vi "Read Values.vi"(8 "error in":errorcluster, 11 "Report Viewer in":refnum<class "Report Viewer.lvclass">) -> (0 "error out":errorcluster, 3 "Report Viewer out":refnum<class "Report Viewer.lvclass">)   [LabVIEW 2019, in "Report Viewer.lvlib" / "Report Viewer.lvclass"]
uses:
  Library/Report Viewer.lvclass
  Library/Report Viewer.lvclass/Report Viewer.ctl
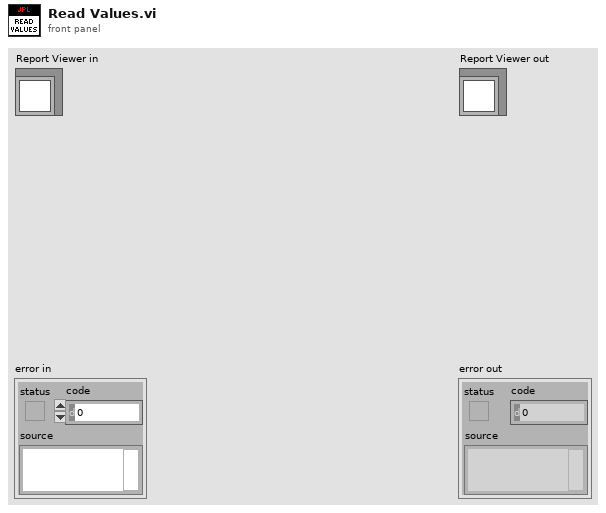
[diagram p1: front panel]
types:
  T1 = typedef "Report Viewer.lvlib/Report Viewer.lvclass/Data to Read.ctl" = cluster{"Group":string, "Channel":string}
  T2 = typedef "Report Viewer.lvlib/Report Viewer.lvclass/Load Method.ctl" = enum16{"Number of Values", "By Time"}
  T3 = typedef "Report Viewer.lvlib/Report Viewer.lvclass/Channel_Timing.ctl" = cluster{"Data Type":u16, "Channel Length":u64, "wf_start_time":timestamp, "wf_increment":dbl}
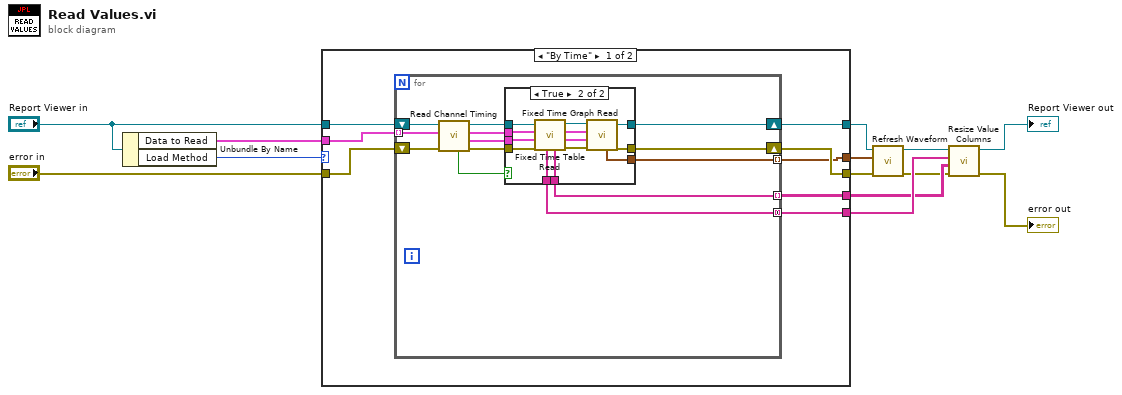
[diagram p0: block diagram]
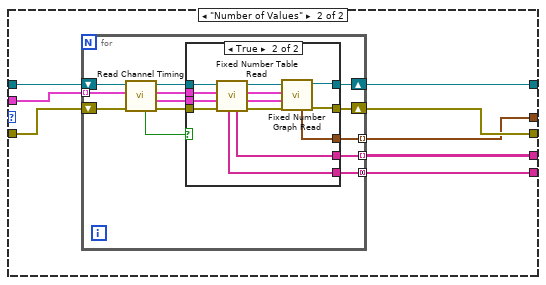
[diagram p3: hidden frame]
diagram:
  n1 = Unbundle By Name("Report Viewer in") -> ("Data to Read"=w9:T1[], "Load Method"=w8:T2)
  n2 = case shown="\"By Time\"" w8 {
    tunnel: [w21 w52] -> w2
    tunnel: [w20 w51] -> w3
    tunnel: "error in" -> [w19 w57]
    tunnel: "Report Viewer in" -> [w18 w56]
    tunnel: w9 -> [w17 w55]
    tunnel: [w15 w54] -> w6
    tunnel: [w16 w53] -> w7
    tunnel: [w14 w50] -> w1
    frame "By Time" {
      n3 = for {
        shift-right: [w34] -> w21
        shift-left: w18 -> [w32]
        shift-right: [w33] -> w20
        shift-left: w19 -> [w28]
        tunnel: w17 -> [w27] mode=indexing
        tunnel: [w24] -> w16 mode=concatenating
        tunnel: [w23] -> w15 mode=indexing
        tunnel: [w22] -> w14 mode=indexing
        n4 = call "Read Channel Timing.vi"("error in"=w28, "Data to read in"=w27, "Report Viewer in"=w32) -> ("error out"=w30:errorcluster, "Data to read out"=w25:T1, "Channel_Timing"=w29:T3, "Report Viewer out"=w31:refnum<class "Report Viewer.lvclass">, "Good_Record"=w26:bool)  [unwired: 4 in]
        n5 = case shown="True" w26 {
          tunnel: [w35 w40] -> w34
          tunnel: [w36 w41] -> w33
          tunnel: w31 -> [w35 w49]
          tunnel: w30 -> [w36 w48]
          tunnel: w29 -> [_ w47]
          tunnel: w25 -> [_ w46]
          tunnel: [_ w45] -> w24
          tunnel: [_ w44] -> w23
          tunnel: [_ w37] -> w22
          frame False {
          }
          frame True {
            n6 = call "Fixed Time Table Read.vi"("error in"=w48, "Data to read in"=w46, "Channel_Timing in"=w47, "Report Viewer in"=w49) -> ("error out"=w42:errorcluster, "Data to read out"=w38:T1, "Channel_Timing out"=w39:T3, "Report Viewer out"=w43:refnum<class "Report Viewer.lvclass">, "Table Data"=w44:string[], "Table_Header"=w45:string[])  [unwired: 2 in]
            n7 = call "Fixed Time Graph Read.vi"("error in"=w42, "Data to read in"=w38, "Channel_Timing in"=w39, "Report Viewer in"=w43) -> ("error out"=w41:errorcluster, "Report Viewer out"=w40:refnum<class "Report Viewer.lvclass">, "Waveform"=w37:waveform(dbl))  [unwired: 3 in, 2 out]
          }
        }
      }
    }
    frame "Number of Values" {
      n8 = for {
        shift-right: [w65] -> w52
        shift-left: w56 -> [w70]
        shift-right: [w64] -> w51
        shift-left: w57 -> [w69]
        tunnel: w55 -> [w68] mode=indexing
        tunnel: [w60] -> w54 mode=indexing
        tunnel: [w59] -> w53 mode=concatenating
        tunnel: [w58] -> w50 mode=indexing
        n9 = call "Read Channel Timing.vi"("error in"=w69, "Data to read in"=w68, "Report Viewer in"=w70) -> ("error out"=w67:errorcluster, "Data to read out"=w61:T1, "Channel_Timing"=w63:T3, "Report Viewer out"=w66:refnum<class "Report Viewer.lvclass">, "Good_Record"=w62:bool)  [unwired: 4 in]
        n10 = case shown="True" w62 {
          tunnel: w67 -> [w71 w81]
          tunnel: w66 -> [w72 w80]
          tunnel: [w72 w84] -> w65
          tunnel: [w71 w85] -> w64
          tunnel: w63 -> [_ w79]
          tunnel: w61 -> [_ w78]
          tunnel: [_ w75] -> w60
          tunnel: [_ w74] -> w59
          tunnel: [_ w73] -> w58
          frame False {
          }
          frame True {
            n11 = call "Fixed Number Table Read.vi"("error in"=w81, "Data to read in"=w78, "Channel_Timing in"=w79, "Report Viewer in"=w80) -> ("error out"=w82:errorcluster, "Data to read out"=w77:T1, "Channel_Timing out"=w76:T3, "Report Viewer out"=w83:refnum<class "Report Viewer.lvclass">, "Table Data"=w75:string[], "Table_Header"=w74:string[])  [unwired: 2 in]
            n12 = call "Fixed Number Graph Read.vi"("error in"=w82, "Data to read in"=w77, "Channel_Timing in"=w76, "Report Viewer in"=w83) -> ("error out"=w85:errorcluster, "Report Viewer out"=w84:refnum<class "Report Viewer.lvclass">, "Waveform"=w73:waveform(dbl))  [unwired: 3 in, 2 out]
          }
        }
      }
    }
  }
  n13 = call "Refresh Waveform.vi"("error in"=w3, "Waveform"=w1, "Report Viewer in"=w2) -> ("error out"=w4:errorcluster, "Report Viewer out"=w5:refnum<class "Report Viewer.lvclass">)  [unwired: 7 in]
  n14 = call "Resize Value Columns.vi"("error in"=w4, "Item Names"=w6, "Column Header"=w7, "Report Viewer in"=w5) -> ("error out"=→"error out":errorcluster, "Report Viewer out"=→"Report Viewer out":refnum<class "Report Viewer.lvclass">)  [unwired: 6 in]
